vi "IMAQDevice.setJPGMode.vi"(0 "i ref in":refnum<vi>, 2 "JPEG Mode?":bool, 5 "error in (no error)":errorcluster) -> (14 "i ref out":refnum<vi>, 19 "error out":errorcluster)   [LabVIEW 2014, in "IMAQDevice.lvlib"]
doc: "This VI allows to reset the mode of the data transfer from normal mode (0) to JPEG mode (1) and vise versa.\n\nLicense Agreement for this software:\n\nCopyright (C)\nGesellschaft für Schwerionenforschung, GSI\nPlanckstr. 1\n64291 Darmstadt\nGermany\n\nContact: D.Beck@gsi.de \n\nThis program is free software; you can redistribute it and/or modify it under the terms of the \nGNU General Public License as published by the Free Software Foundation; either version 2 of \nthe license, or (at your option) any later version.\n\nThis program is distributed in the hope that it will be useful, but WITHOUT ANY WARRANTY; \nwithout even the implied warranty of MERCHANTABILITY or FITNESS FOR A PARTICULAR PURPOSE. See the GNU General License for more details (http://www.gnu.org).\n\nGesellschaft für Schwerionenforschung, GSI\nPlanckstr. 1, 64291 Darmstadt, Germany\nFor all questions and ideas contact: M.Richter@gsi.de, H.Brand@gsi.de or D.Beck@gsi.de.\nLast update: 16-JUN-2004"
uses:
  IMAQDevice.lvlib
  CSlibraries-extern/DimLVEvent/LVDimInterface/LVDimInterface.lvlib
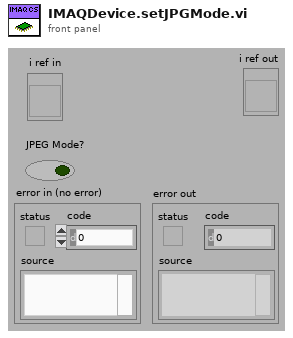
[diagram p1: front panel]
types:
  T1 = typedef "IMAQDevice.lvlib/IMAQDevice.i attribute.ctl" = cluster{"HGF_IMAQ.lvlib:HGF_IMAQDevice.lvclass":refnum<class "HGF_IMAQDevice.lvclass">, "Image":T2, "TimeStampID":i32, "Image IDs":i32[], "NumberOfImagesID":i32, "JPEG?":bool, "JPEGID":i32, "JPEG_ImageID":i32, "TriggerModeID":i32, "OffsetFromLeft":i32, "OffsetFromTop":i32, "HorizontalPixelPerMm":dbl, "VerticalPixelPerMm":dbl, "Grid":cluster{"1":cluster{i32, i32}, "2":cluster{i32, i32}, "3":cluster{i32, i32}, "4":cluster{i32, i32}}, "GridR":cluster{"1":cluster{dbl, dbl}, "2":cluster{dbl, dbl}, "3":cluster{dbl, dbl}, "4":cluster{dbl, dbl}}, "CameraTypeID":i32, "CameraInfos":cluster{"Camera Name-Array":string[], "own Camera Type":string}, "TakeMeasurement?":bool, "TriggerArmedID":i32, "Mirroring":i16, "Rotation":dbl}
  T2 = typedef "IMAQ Image.ctl" = refnum<image>
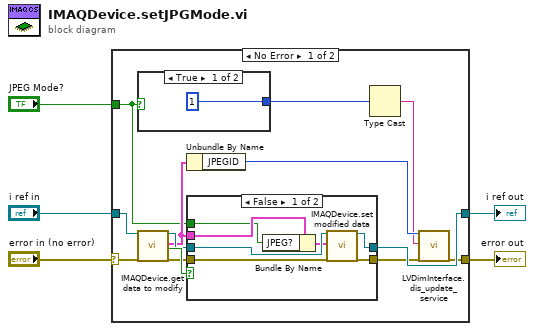
[diagram p0: block diagram]
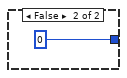
[diagram p2: hidden frame]
diagram:
  n1 = case shown="No Error" "error in (no error)" {
    selector: "error in (no error)" -> [w17 w31]
    tunnel: "i ref in" -> [w18 w30]
    tunnel: [w11 w31] -> w3
    tunnel: [w15 w30] -> w2
    tunnel: "JPEG Mode?" -> [w6 _]
    frame No Error {
      n2 = case shown="True" w6 {
        tunnel: [i16 1 ("x") i16 0 ("x")] -> w8
        frame True {
        }
        frame False {
        }
      }
      n3 = call "IMAQDevice.get data to modify.vi"("i ref in"=w18, "error in (no error)"=w17) -> ("i ref out"=w14:refnum<vi>, "i attribute"=w10:T1, "timed out"=w16:bool, "error out"=w13:errorcluster)  [unwired: 14 in]
      n4 = Unbundle By Name(w10) -> ("JPEGID"=w9:i32)
      n5 = case shown="False" w16 {
        tunnel: [w27 w29] -> w15
        tunnel: w14 -> [w26 w29]
        tunnel: w13 -> [w25 w28]
        tunnel: [w24 w28] -> w12
        tunnel: w10 -> [w23 _]
        tunnel: w6 -> [w22 _]
        frame False {
          n6 = Bundle By Name(cluster=w23, "JPEG?"=w22) -> (w21:T1)
          n7 = call "IMAQDevice.set modified data.vi"("i ref in"=w26, "i attribute"=w21, "error in (no error)"=w25) -> ("i ref out"=w27:refnum<vi>, "error out"=w24:errorcluster)  [unwired: 15 in]
        }
        frame True {
        }
      }
      n8 = Type Cast(x=w8) -> (*(type *) &x=w7:string)  [unwired: 1 in]
      n9 = call "LVDimInterface.dis_update_service.vi"("my_serviceID"=w9, "data"=w7, "error in (no error)"=w12) -> ("error out"=w11:errorcluster)  [unwired: 14 in, 2 out]
    }
    frame Error {
    }
  }
  "i ref out" <- w2
  "error out" <- w3
